vi "Grab.vi"(8 "error in (no error)":errorcluster, 11 "reference in":refnum<class "Camera_IMAQdx.lvclass">) -> (0 "error out":errorcluster, 1 "Frame Number":u32, 2 "Image Out":T1, 3 "reference out":refnum<class "Camera_IMAQdx.lvclass">)   [LabVIEW 2017, in "Camera_IMAQdx.lvclass"]
doc: "Grabs the latest image in the image buffer for an acquisition that has been started. Must be used with Start and StopAcquisition."
uses:
  Camera_IMAQdx.lvclass
  <vilib>/vision/driver/NI_Vision_Acquisition_Software.lvlib
  <vilib>/vision/Image Controls.llb/IMAQ Image.ctl
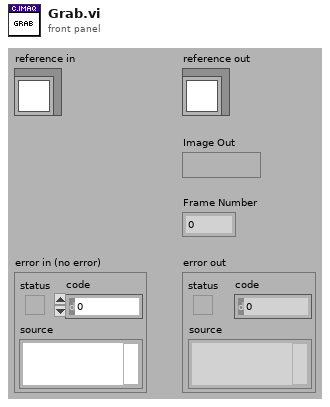
[diagram p1: front panel]
types:
  T1 = typedef "IMAQ Image.ctl" = refnum<image>
  T2 = typedef "IMAQdx.ctl" = refnum<k21>
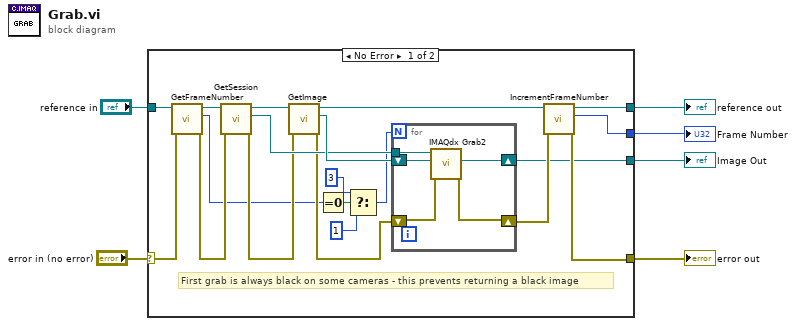
[diagram p0: block diagram]
diagram:
  n1 = case shown="No Error" "error in (no error)" {
    selector: "error in (no error)" -> [w13 w33]
    tunnel: [w18 w33] -> w5
    tunnel: [w20 w32] -> w3
    tunnel: "reference in" -> [w26 w32]
    tunnel: [w16 _] -> w1
    tunnel: [w15 _] -> w2
    frame No Error {
      # "First grab is always black on some cameras - this prevents returning a black image"
      n2 = call-dynamic "GetFrameNumber.vi"("error in (no error)"=w13, "reference in"=w26) -> ("error out"=w12:errorcluster, "Grab Frame Number"=w11:u32, "reference in"=w14:refnum<class "Camera_IMAQdx.lvclass">)  [unwired: 7 in]
      n3 = call "GetSession.vi"("error in (no error)"=w12, "reference in"=w14) -> ("error out"=w22:errorcluster, "Session"=w23:T2, "reference out"=w25:refnum<class "Camera_IMAQdx.lvclass">)  [unwired: 7 in]
      n4 = call "GetImage.vi"("error in (no error)"=w22, "reference in"=w25) -> ("error out"=w19:errorcluster, "Image"=w24:T1, "reference out"=w21:refnum<class "Camera_IMAQdx.lvclass">)  [unwired: 7 in]
      n5 = Equal To 0?(x=w11) -> (x = 0?=w10:bool)
      n6 = Select(t=3, s=w10, f=1) -> (s? t:f=w7:i32)
      n7 = for {
        N: w7 -> [_]
        tunnel: w23 -> [w30]
        shift-right: [w27] -> w16
        shift-left: w24 -> [w31]
        shift-right: [w28] -> w17
        shift-left: w19 -> [w29]
        n8 = call <vilib>:"IMAQdx Grab2.vi"("error in"=w29, "Image In"=w31, "Session In"=w30) -> ("error out"=w28:errorcluster, "Image Out"=w27:T1)  [unwired: 5 in, 2 out]
      }
      n9 = call "IncrementFrameNumber.vi"("error in (no error)"=w17, "reference in"=w21) -> ("error out"=w18:errorcluster, "Frame Number"=w15:u32, "reference out"=w20:refnum<class "Camera_IMAQdx.lvclass">)  [unwired: 7 in]
    }
    frame Error {
    }
  }
  "error out" <- w5
  "reference out" <- w3
  "Image Out" <- w1
  "Frame Number" <- w2
